vi "AutoFireStateMachine.vi"(7 "FrisbeeInChamber":bool, 8 "AutoFire":bool, 9 "TriggerPulled":bool, 10 "LastShotComplete":bool, 11 "LastState":enum16{"Ready", "Fire1", "Auto"}(ring)) -> (1 "SolenoidState":T1, 2 "ShotComplete":bool, 3 "NextState":enum16{"Ready", "Fire1", "Auto"}(ring))   [LabVIEW 2012]
uses:
  <vilib>/Rock Robotics/WPI/Solenoid/WPI_SolenoidValue.ctl
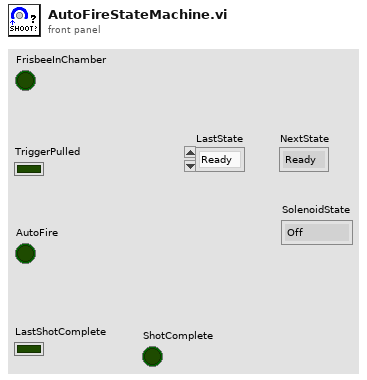
[diagram p1: front panel]
types:
  T1 = typedef "WPI_SolenoidValue.ctl" = enum16{"Off", "On", "Forward", "Reverse"}
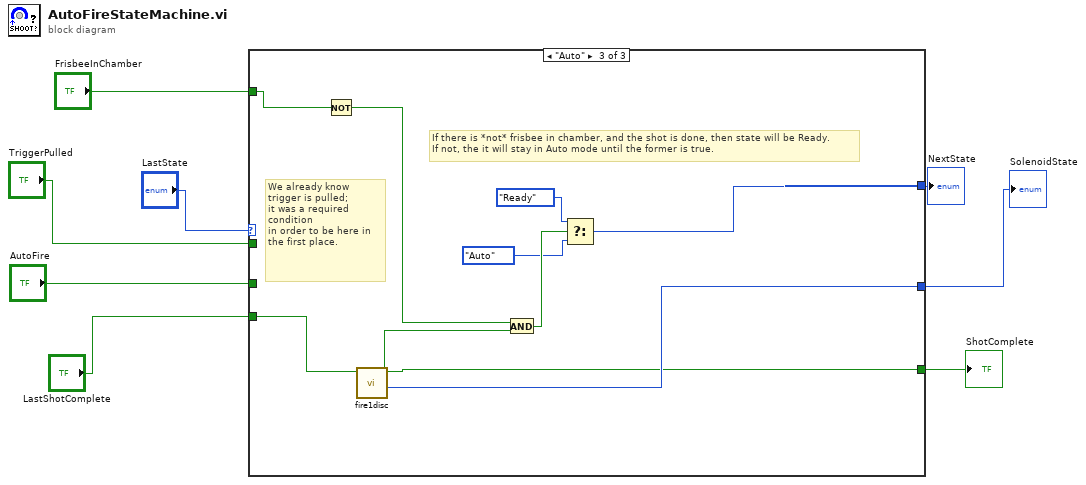
[diagram p0: block diagram]
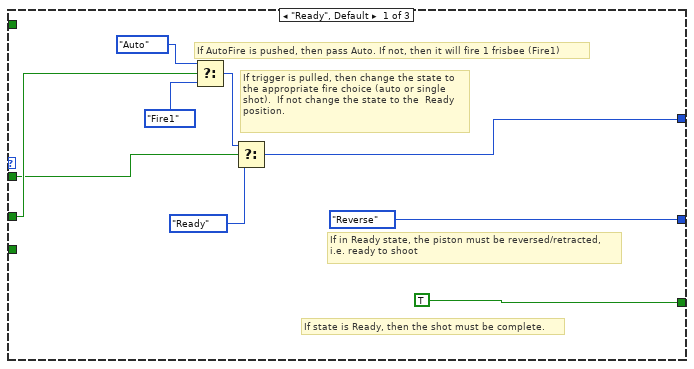
[diagram p2: hidden frame]
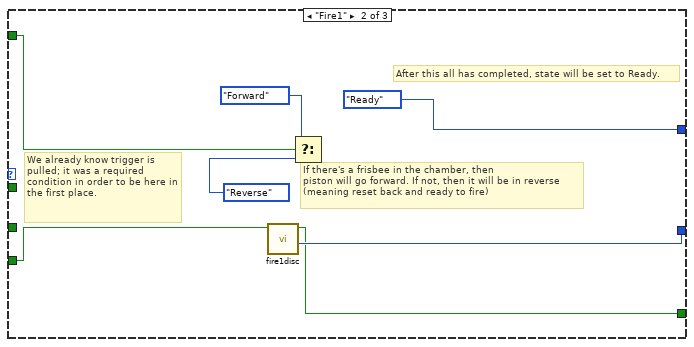
[diagram p3: hidden frame]
diagram:
  n1 = case shown="\"Auto\"" "LastState" {
    tunnel: "FrisbeeInChamber" -> [_ w24 w28]
    tunnel: "TriggerPulled" -> [w12 _ _]
    tunnel: [w11 enum16{"Ready", "Fire1", "Auto"}."Ready" w30] -> w4
    tunnel: "AutoFire" -> [w13 _ _]
    tunnel: [WPI_SolenoidValue."Reverse" ("SolenoidState 2") w20 w29] -> w3
    tunnel: "LastShotComplete" -> [_ w18 w26]
    tunnel: [TRUE w19 w25] -> w1
    frame "Ready", Default {
      # "If AutoFire is pushed, then pass Auto. If not, then it will fire 1 frisbee (Fire1)"
      # "If trigger is pulled, then change the state to the appropriate fire choice (auto or single shot).  If not change the state to the  Ready position."
      # "If in Ready state, the piston must be reversed/retracted,\ni.e. ready to shoot"
      # "If state is Ready, then the shot must be complete."
      n2 = Select(t=enum16{"Ready", "Fire1", "Auto"}."Auto", s=w13, f=enum16{"Ready", "Fire1", "Auto"}."Fire1") -> (s? t:f=w16:enum16{"Ready", "Fire1", "Auto"})
      n3 = Select(t=w16, s=w12, f=enum16{"Ready", "Fire1", "Auto"}."Ready") -> (s? t:f=w11:enum16{"Ready", "Fire1", "Auto"})
    }
    frame "Fire1" {
      # "After this all has completed, state will be set to Ready."
      # "If there's a frisbee in the chamber, then\npiston will go forward. If not, then it will be in reverse\n(meaning reset back and ready to fire)"
      # "We already know trigger is pulled; it was a required\ncondition in order to be here in the first place."
      n4 = call "fire1disc.vi"("Reset Count"=w18) -> ("Launcher State"=w20:T1, "Done"=w19:bool)  [unwired: 9 in]
      n5 = Select(t=WPI_SolenoidValue."Forward" ("SolenoidState 2"), s=w24, f=WPI_SolenoidValue."Reverse" ("SolenoidState 2")) -> ()  [unwired: 1 out]
    }
    frame "Auto" {
      # "If there is *not* frisbee in chamber, and the shot is done, then state will be Ready.\nIf not, the it will stay in Auto mode until the former is true."
      # "We already know trigger is pulled; \nit was a required condition\nin order to be here in the first place."
      n6 = Not(x=w28) -> (.not. x?=w27:bool)
      n7 = call "fire1disc.vi"("Reset Count"=w26) -> ("Launcher State"=w29:T1, "Done"=w25:bool)  [unwired: 9 in]
      n8 = And(x=w27, y=w25) -> (x .and. y?=w33:bool)
      n9 = Select(t=enum16{"Ready", "Fire1", "Auto"}."Ready", s=w33, f=enum16{"Ready", "Fire1", "Auto"}."Auto") -> (s? t:f=w30:enum16{"Ready", "Fire1", "Auto"})
    }
  }
  "SolenoidState" <- w3
  "NextState" <- w4
  "ShotComplete" <- w1
